vi "Toggle Mode.vi"(11 "Toggle":bool) -> ()   [LabVIEW 2012]
panel:
  out "Middle Mode":bool=TRUE
  out "Outer Mode":bool=TRUE
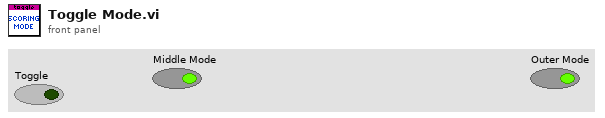
[diagram p1: front panel]
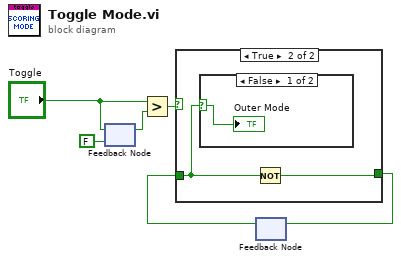
[diagram p0: block diagram]
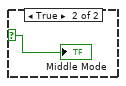
[diagram p3: hidden frame]
diagram:
  n1 = feedback #1(FALSE ("Button 11")) -> (w5:bool)
  n2 = feedback-in #1("Toggle") -> ()
  n3 = Greater?(x="Toggle", y=w5) -> (0:w3:bool)
  n4 = feedback #2() -> (w1:bool)  [unwired: 1 in]
  n5 = case shown="True" w3 {
    tunnel: [w7 w9] -> w2
    tunnel: w1 -> [w7 w8]
    frame False {
    }
    frame True {
      n6 = case shown="False" w8 {
        selector: w8 -> [w10 w11]
        frame False {
          "Outer Mode" <- w10
        }
        frame True {
          "Middle Mode" <- w11
        }
      }
      n7 = Not(x=w8) -> (.not. x?=w9:bool)
    }
  }
  n8 = feedback-in #2(w2) -> ()
